vi "read_status.vi"(8 "error in (no error)":errorcluster, 11 "VISA resource name":refnum<visa-resource-name>) -> (0 "error out":errorcluster, 2 "Status cluster":T1, 3 "VISA resource name out":refnum<visa-resource-name>)   [LabVIEW 2018]
uses:
  status_cluster.ctl
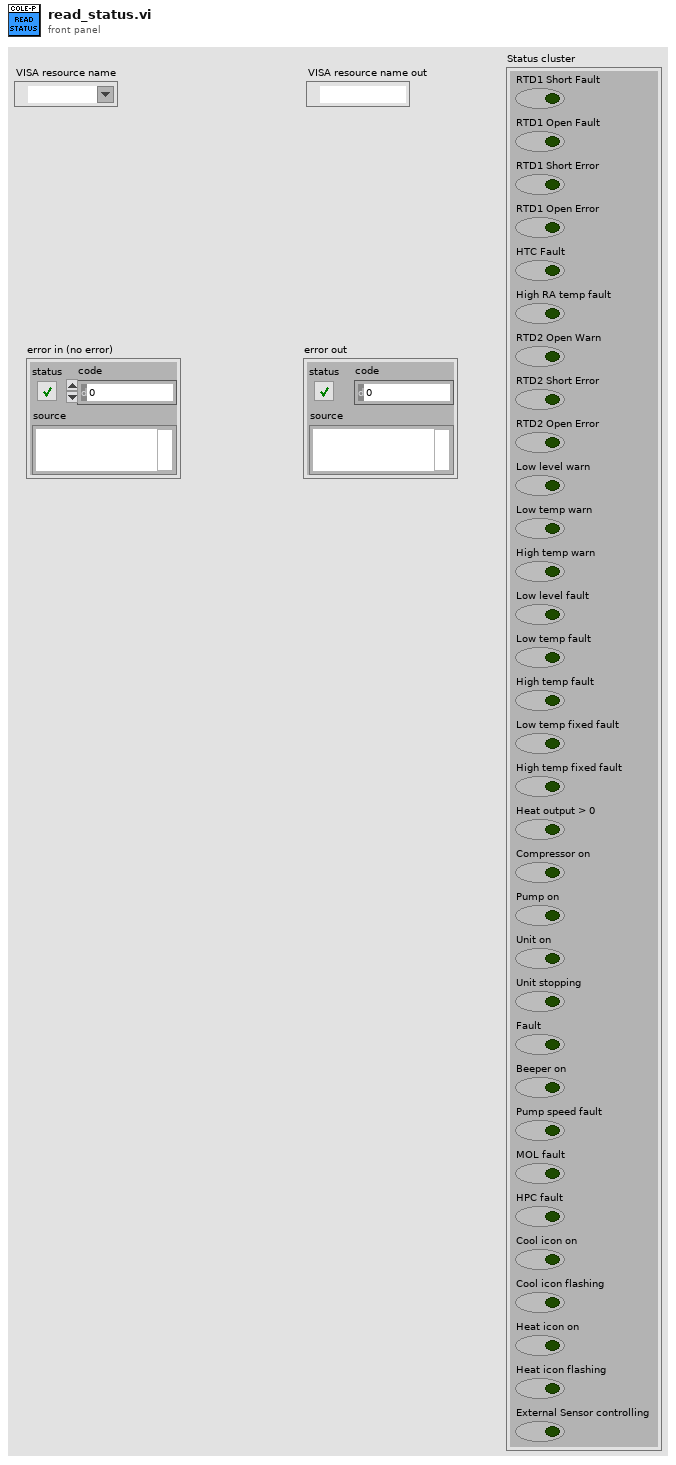
[diagram p1: front panel]
types:
  T1 = typedef "status_cluster.ctl" = cluster{"RTD1 Short Fault":bool, "RTD1 Open Fault":bool, "RTD1 Short Error":bool, "RTD1 Open Error":bool, "HTC Fault":bool, "High RA temp fault":bool, "RTD2 Open Warn":bool, "RTD2 Short Error":bool, "RTD2 Open Error":bool, "Low level warn":bool, "Low temp warn":bool, "High temp warn":bool, "Low level fault":bool, "Low temp fault":bool, "High temp fault":bool, "Low temp fixed fault":bool, "High temp fixed fault":bool, "Heat output > 0":bool, "Compressor on":bool, "Pump on":bool, "Unit on":bool, "Unit stopping":bool, "Fault":bool, "Beeper on":bool, "Pump speed fault":bool, "MOL fault":bool, "HPC fault":bool, "Cool icon on":bool, "Cool icon flashing":bool, "Heat icon on":bool, "Heat icon flashing":bool, "External Sensor controlling":bool}
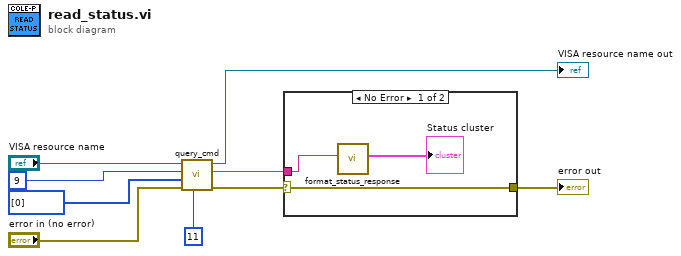
[diagram p0: block diagram]
diagram:
  n1 = call "query_cmd.vi"("Number of bytes in response"=u32 11, "error in (no error)"="error in (no error)", "Data bytes"=u8[] [0], "Command byte"=u8 9, "VISA resource name"="VISA resource name") -> ("error out"=w2:errorcluster, "Response"=w3:string, "VISA resource name out"=→"VISA resource name out":refnum<visa-resource-name>)  [unwired: 4 in]
  n2 = case shown="No Error" w2 {
    selector: w2 -> [w12 w13]
    tunnel: w3 -> [w11 _]
    tunnel: [w12 w13] -> w1
    frame No Error {
      n3 = call "format_status_response.vi"("Response"=w11) -> ("Status cluster"=→"Status cluster":T1)  [unwired: 10 in]
    }
    frame Error {
    }
  }
  "error out" <- w1
